vi "1D_Plot.ly_Ex.vi"() -> ()   [LabVIEW 2025]
doc: "Demonstrates how to write a simple 1D array to Plot.ly."
uses:
  <vilib>/Foerster.tech/LabPlot.ly/LabPlot.ly/Typdef/graphSettings.ctl
  <vilib>/Foerster.tech/LabPlot.ly/LabPlot.ly/Typdef/mode.ctl
  <vilib>/Foerster.tech/LabPlot.ly/LabPlot.ly/Typdef/line.ctl
  <vilib>/Foerster.tech/LabPlot.ly/LabPlot.ly/Typdef/dash.ctl
  <vilib>/Foerster.tech/LabPlot.ly/LabPlot.ly/LabPlot.ly.lvlib
  <vilib>/Analysis/NI_AALBase.lvlib
panel:
  out "File Path out":path
  out "Execution Time[ms]":u32
  in  "cycles":dbl=5.0 format="%0.2f"
  out "Waveform Graph":dbl[](graph)
  in  "Call Setup":bool
  in  "graphSettings":T1={"mode"=enum."lines+markers", "line"={"color"=44543, "width"=2, "dash"=enum."solid"}}
  in  "File Path Control(empty: only show graph)":path
  in  "Reduction(0: No Reduction)":i32
  in  "amplitude":dbl=5.0 format="%0.2f"
  in  "samples":i32=50000
  # "Sinewave Settings"
  # "Call asynchronously to not hold up your program"
  # "This Program demonstrates how to print a 1D Array to Plot.ly\n\nYou can output the plot to browser without saving it by leaving File Path empty or save the html file by selecting a path.\n\nSince Plot.ly stores the data in the html, plots of >200k points become slow to open. It's recommended you use the built-in Reduction to reduce your dataset."
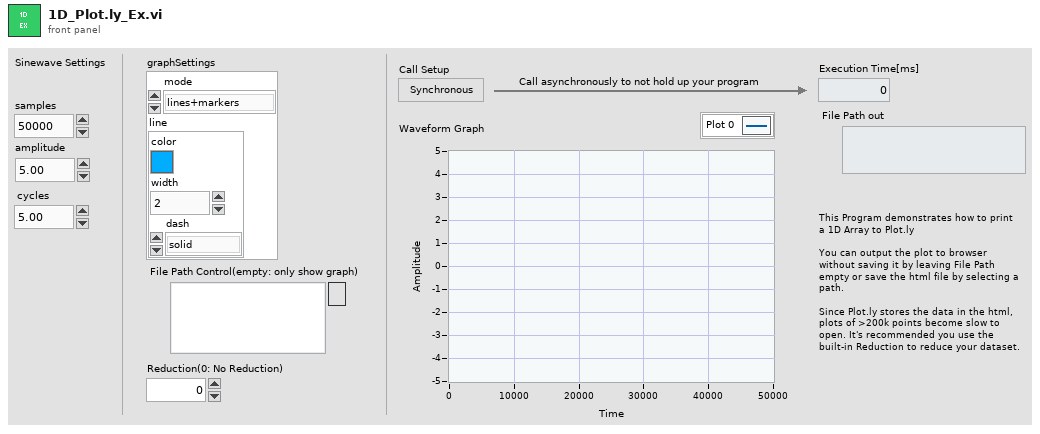
[diagram p1: front panel]
types:
  T1 = typedef "LabPlot.ly.lvlib/graphSettings.ctl" = cluster{"mode":T2, "line":T3}
  T2 = typedef "LabPlot.ly.lvlib/mode.ctl" = enum16{"lines", "markers", "text", "lines+markers", "markers+text", "lines+text", "lines+markers+text"}
  T3 = typedef "LabPlot.ly.lvlib/line.ctl" = cluster{"color":u32, "width":i32, "dash":T4}
  T4 = typedef "LabPlot.ly.lvlib/dash.ctl" = enum16{"solid", "dot", "dash", "longdash", "dashdot", "longdashdot"}
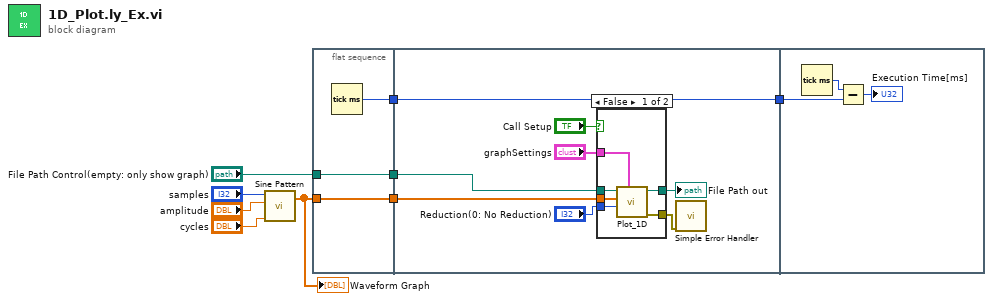
[diagram p0: block diagram]
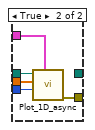
[diagram p2: hidden frame]
diagram:
  n1 = call <vilib>:"Sine Pattern.vi"("cycles"="cycles", "amplitude"="amplitude", "samples"="samples") -> ("Sinusoidal Pattern"=w2:dbl[])  [unwired: 1 in, 1 out]
  "Waveform Graph" <- w2
  n2 = flat-sequence {
    tunnel: "File Path Control(empty: only show graph)" -> [w12]
    tunnel: [w12] -> w8
    tunnel: [w11] -> w7
    tunnel: w2 -> [w10]
    tunnel: [w10] -> w3
    tunnel: w8 -> [w19]
    tunnel: w7 -> [w16]
    tunnel: [w16] -> w6
    tunnel: w3 -> [w15]
    tunnel: w6 -> [w33]
    frame #0 {
      n3 = Tick Count (ms)() -> (millisecond timer value=w11:u32)
    }
    frame #1 {
      n4 = case shown="False" "Call Setup" {
        tunnel: "Reduction(0: No Reduction)" -> [w26 w29]
        tunnel: w19 -> [w25 w31]
        tunnel: "graphSettings" -> [w24 w30]
        tunnel: [w23 w28] -> w13
        tunnel: [w22 _] -> w14
        tunnel: w15 -> [w21 w27]
        frame False {
          n5 = call <vilib>:"Plot_1D.vi"("graphSettings"=w24, "Reduction(0: No Reduction)"=w26, "1D-Data"=w21, "File Path Control(empty: only show graph)"=w25) -> ("Error Out"=w23:errorcluster, "File Path Indicator"=w22:path)  [unwired: 6 in]
        }
        frame True {
          n6 = call <vilib>:"Plot_1D_async.vi"("graphSettings"=w30, "Reduction(0: No Reduction)"=w29, "1D-Data"=w27, "File Path Control(empty: only show graph)"=w31) -> ("Error Out"=w28:errorcluster)  [unwired: 7 in]
        }
      }
      "File Path out" <- w14
      n7 = call <vilib>:"Simple Error Handler.vi"("error in (no error)"=w13) -> ()  [unwired: 4 in, 5 out]
    }
    frame #2 {
      n8 = Tick Count (ms)() -> (millisecond timer value=w34:u32)
      n9 = Subtract(x=w34, y=w33) -> (x-y=→"Execution Time[ms]":u32)
    }
  }
